vi "Create Instrument SMO Name.vi"(8 "error in (no error)":errorcluster, 11 "VoltageUpdate":refnum<class "VoltageUpdate.lvclass">) -> (0 "error out":errorcluster, 2 "SMO Name":string, 3 "VoltageUpdate out":refnum<class "VoltageUpdate.lvclass">)   [LabVIEW 2016, in "VoltageUpdate.lvclass"]
uses:
  VoltageUpdate.lvclass
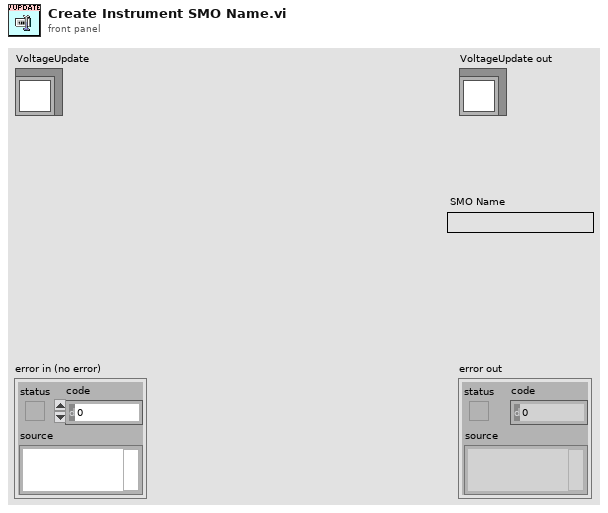
[diagram p1: front panel]
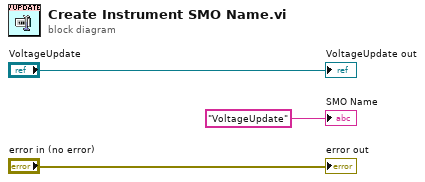
[diagram p0: block diagram]
diagram:
  "error out" <- "error in (no error)"
  "VoltageUpdate out" <- "VoltageUpdate"
  "SMO Name" <- "VoltageUpdate" ("SMO Name")
